vi "GVVentilposition.vi"() -> ()   [LabVIEW 2010, in "Licor-Steuerung.lvlib"]
uses:
  Licor-Steuerung.lvlib
panel:
  in  "Ventilposition":i32=1 min=1 max=6 step=1
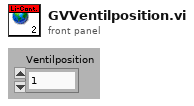
[diagram p1: front panel]
diagram:
